vi "Car Data Live.vi"(1 "Input Array":string[](array[string])) -> (0 "CAR DATA":T1)   [LabVIEW 2014]
uses:
  Type Def/CAR Data Cluster.ctl
  Type Def/CAN Message Live.ctl
panel:
  out "Time Size":i32
  out "Time":dbl[](array[numeric]) format="%.2f"
  out "DECAYIGN(+) - DECAYIGN(-)":dbl
  out "DECAYINJ(+) - DECAYINJ(-)":dbl
  out "DTPS-":dbl
  out "DTPS+":dbl
  out "Speed 2":dbl
  out "Speed 1":dbl
  out "Phase High":dbl
  out "Phase Low":dbl
  out "Spark 1":dbl
  out "Inj Low":dbl
  out "K Lambda 2":dbl
  out "K Lambda 1":dbl
  out "Lambda 2 AVG":dbl
  out "Lambda 2 RAW":dbl
  out "Lambda 1 RAW":dbl
  out "Lambda 1 AVG":dbl
  out "BAR0":u32
  out "VBB 3":dbl
  out "VBB 2":dbl
  out "VBB 1":dbl
  out "T Oil":u32
  out "T Air":i32
  out "T H20":i32
  out "map":u32
  out "TPS":dbl
  out "rev/min":u32
  out "revs":u32
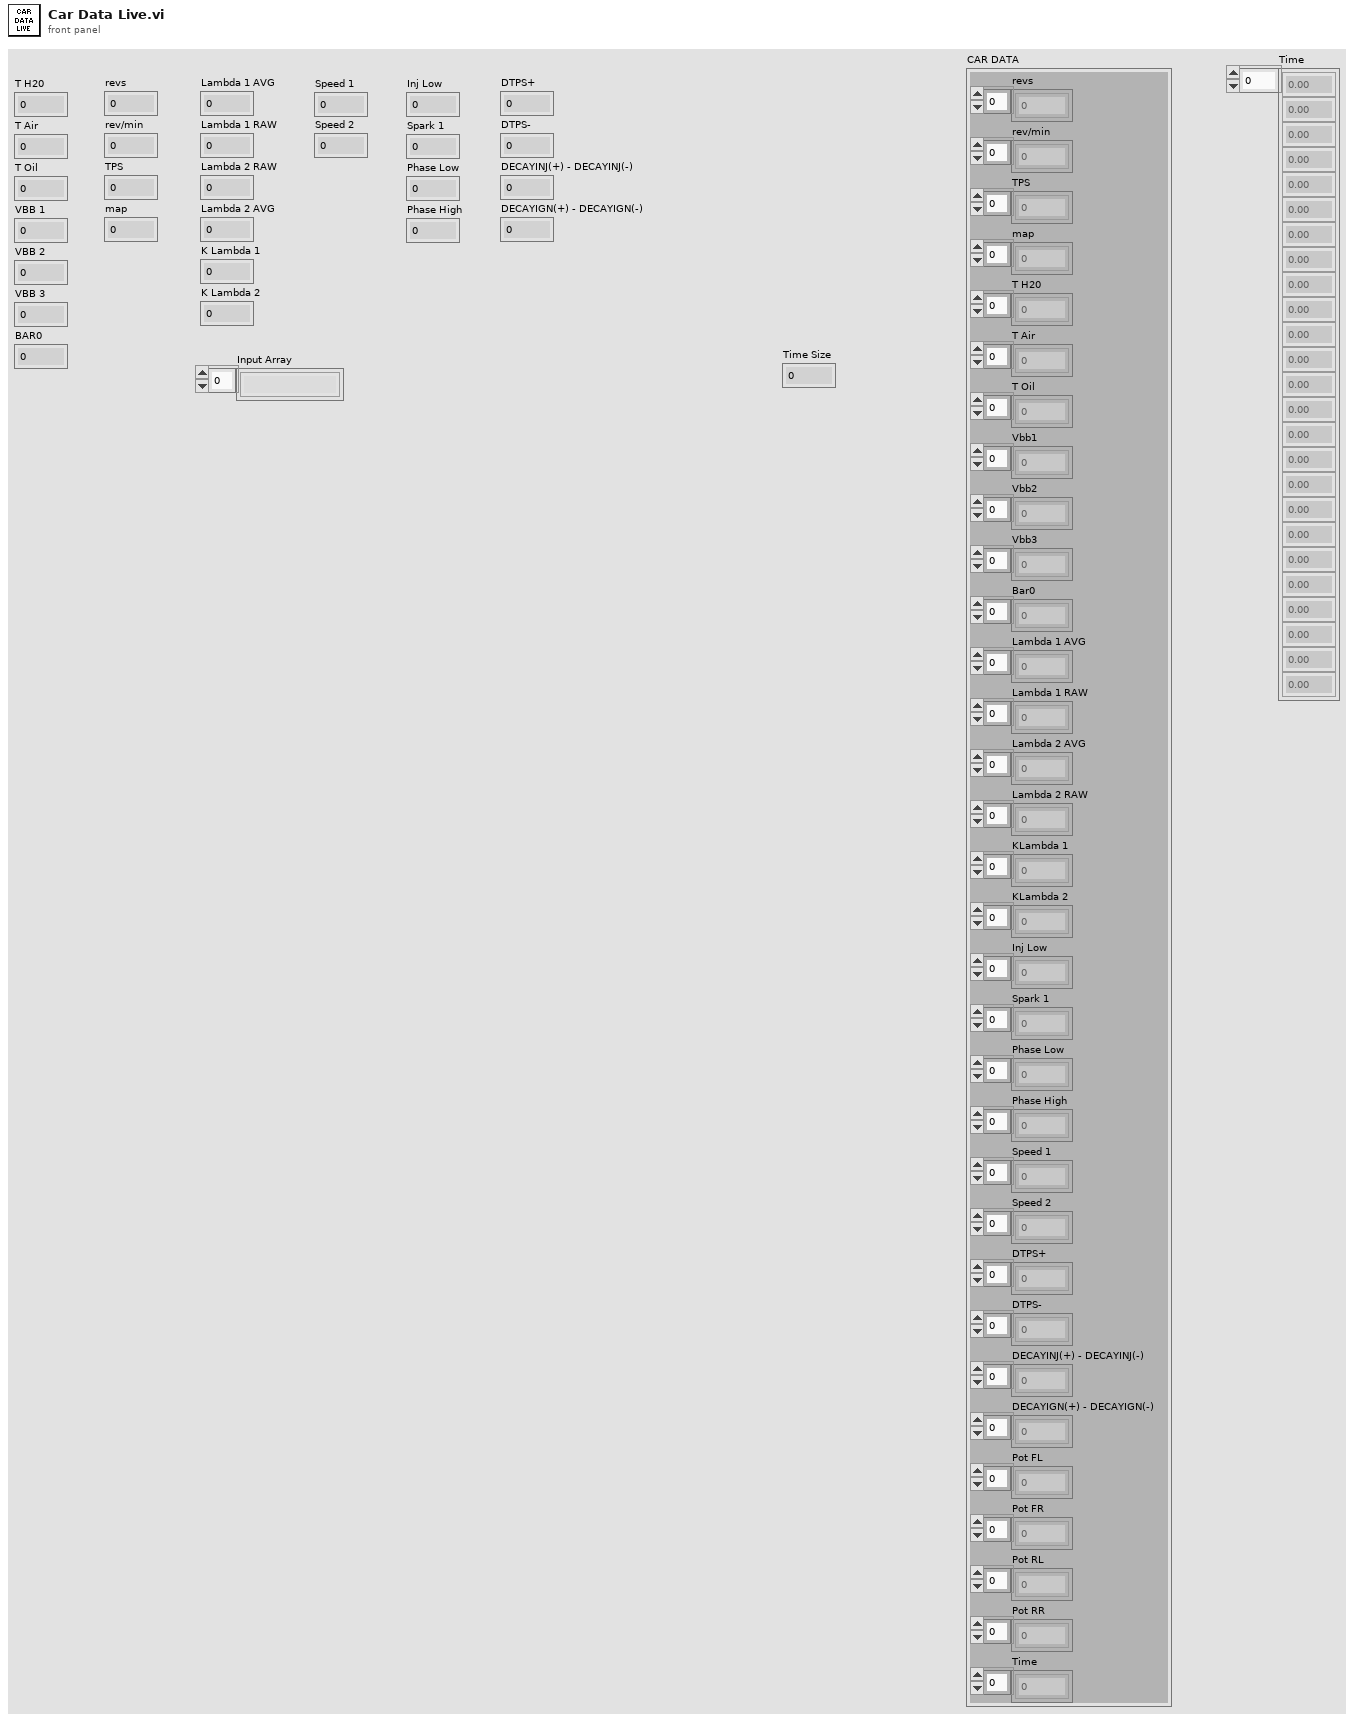
[diagram p1: front panel]
types:
  T1 = typedef "CAR Data Cluster.ctl" = cluster{"revs":dbl[], "rev/min":dbl[], "TPS":dbl[], "map":dbl[], "T H20":dbl[], "T Air":dbl[], "T Oil":dbl[], "Vbb1":dbl[], "Vbb2":dbl[], "Vbb3":dbl[], "Bar0":dbl[], "Lambda 1 AVG":dbl[], "Lambda 1 RAW":dbl[], "Lambda 2 AVG":dbl[], "Lambda 2 RAW":dbl[], "KLambda 1":dbl[], "KLambda 2":dbl[], "Inj Low":dbl[], "Spark 1":dbl[], "Phase Low":dbl[], "Phase High":dbl[], "Speed 1":dbl[], "Speed 2":dbl[], "DTPS+":dbl[], "DTPS-":dbl[], "DECAYINJ(+) - DECAYINJ(-)":dbl[], "DECAYIGN(+) - DECAYIGN(-)":dbl[], "Pot FL":dbl[], "Pot FR":dbl[], "Pot RL":dbl[], "Pot RR":dbl[], "Time":dbl[]}
  T2 = cluster{"revs":dbl[], "rev/min":dbl[], "TPS":dbl[], "map":dbl[], "T H20":dbl[], "T Air":dbl[], "T Oil":dbl[], "Vbb1":dbl[], "Vbb2":dbl[], "Vbb3":dbl[], "Bar0":dbl[], "Lambda 1 AVG":dbl[], "Lambda 1 RAW":dbl[], "Lambda 2 AVG":dbl[], "Lambda 2 RAW":dbl[], "KLambda 1":dbl[], "KLambda 2":dbl[], "Inj Low":dbl[], "Spark 1":dbl[], "Phase Low":dbl[], "Phase High":dbl[], "Speed 1":dbl[], "Speed 2":dbl[], "DTPS+":dbl[], "DTPS-":dbl[], "DECAYINJ(+) - DECAYINJ(-)":dbl[], "DECAYIGN(+) - DECAYIGN(-)":dbl[], "Pot FL":dbl[], "Pot FR":dbl[], "Pot RL":dbl[], "Pot RR":dbl[], "Time":dbl[]}
  T3 = typedef "CAN Message Live.ctl" = cluster{"Time Dif.":i32, "ID":i32, "Message":string}
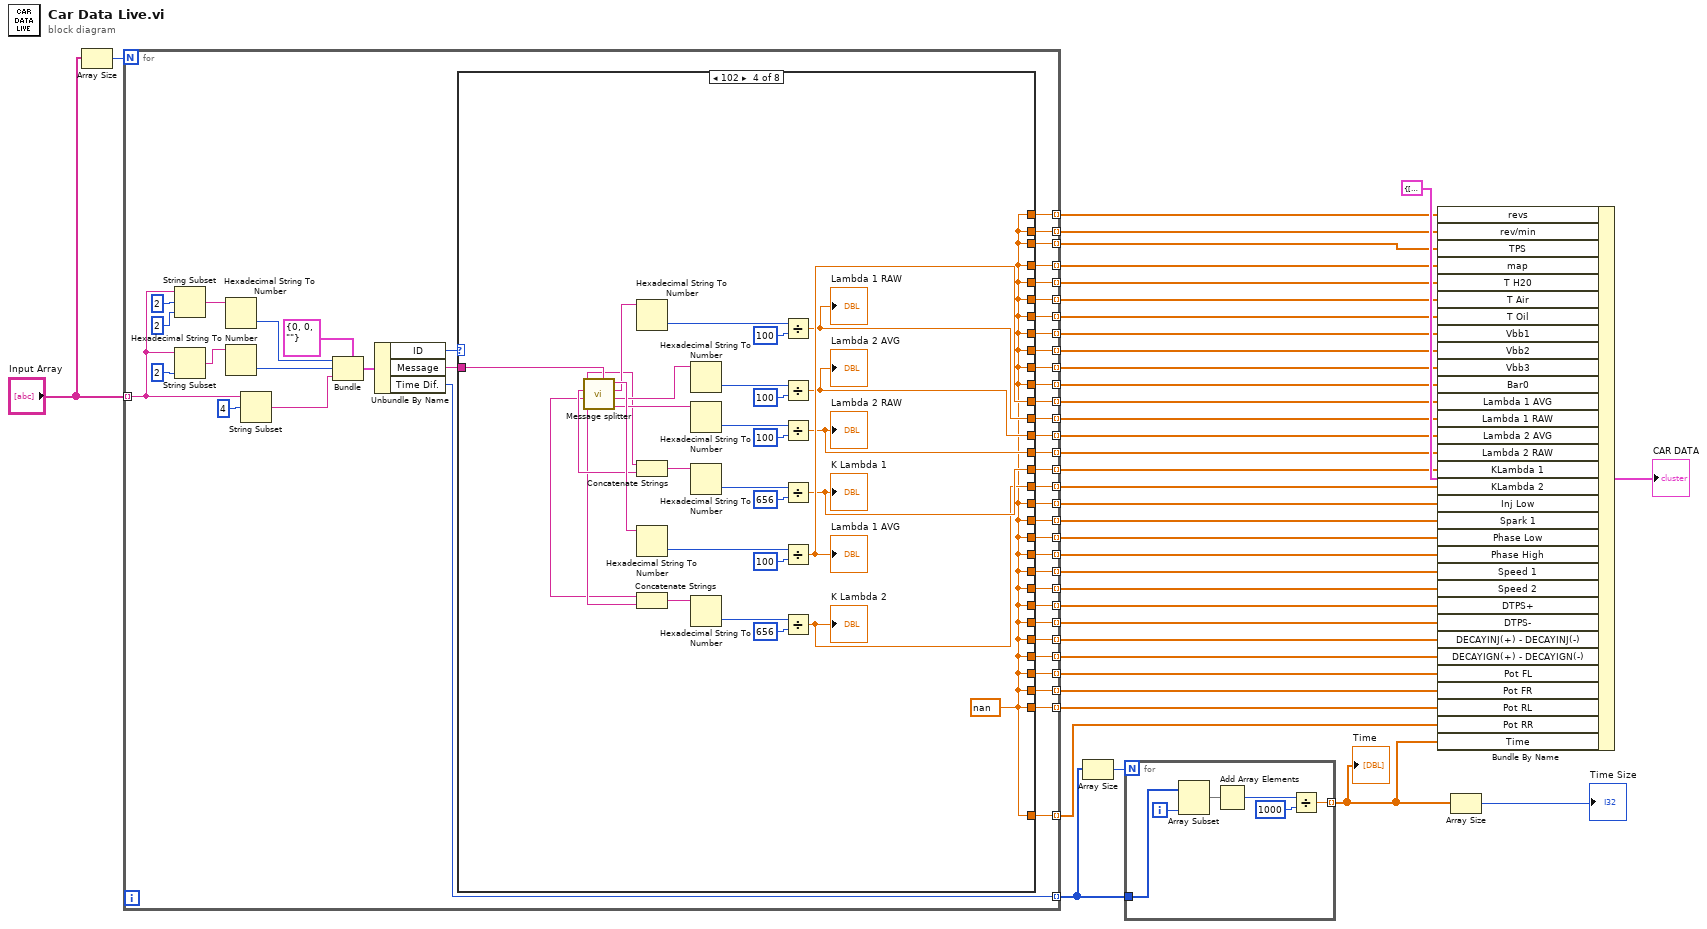
[diagram p0: block diagram]
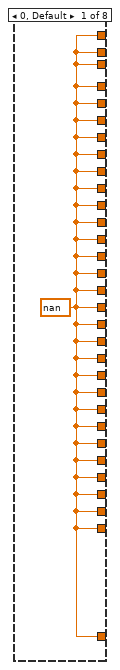
[diagram p2: hidden frame]
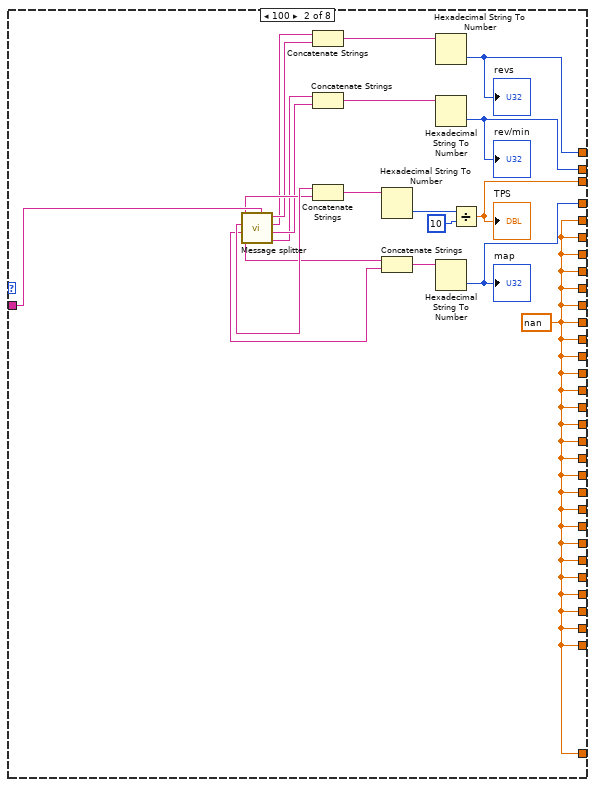
[diagram p3: hidden frame]
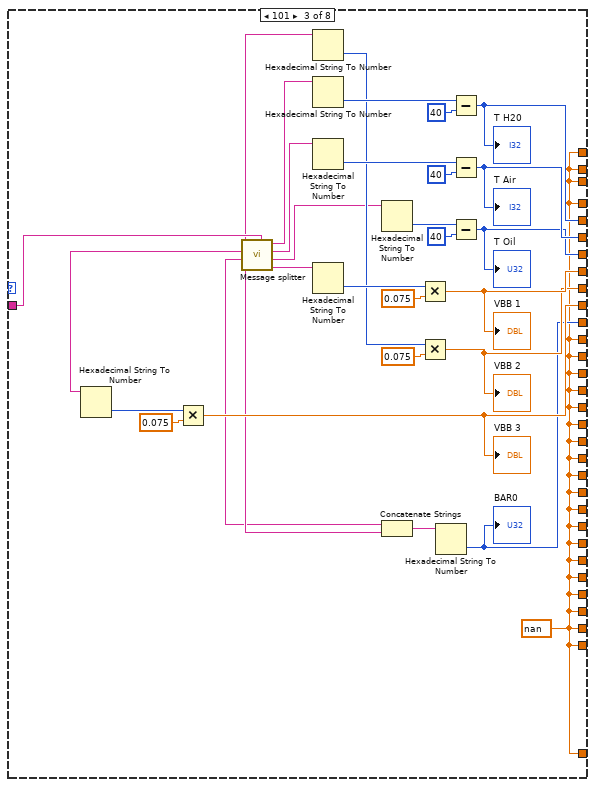
[diagram p4: hidden frame]
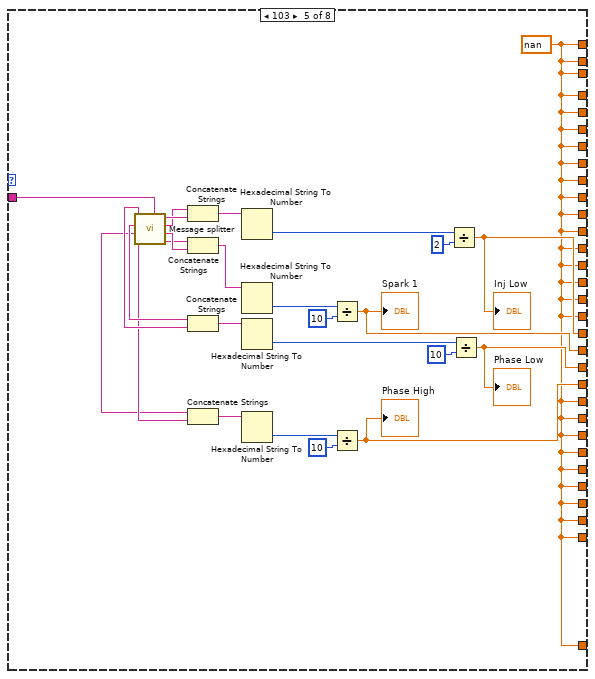
[diagram p5: hidden frame]
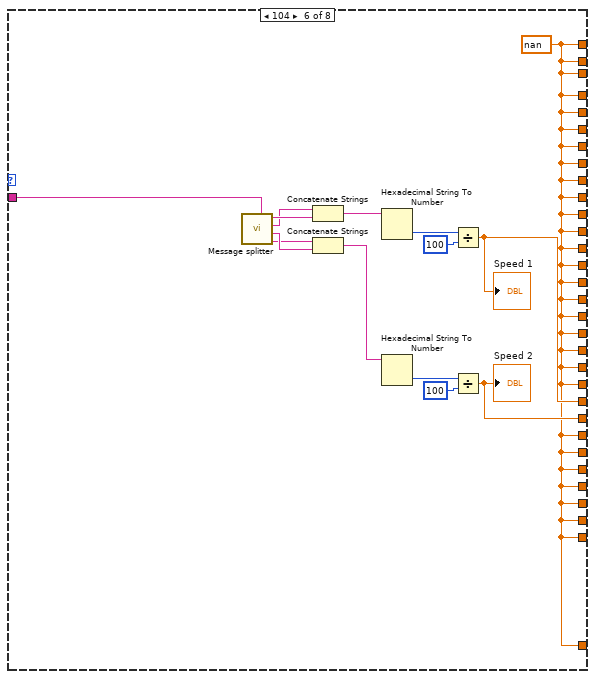
[diagram p6: hidden frame]
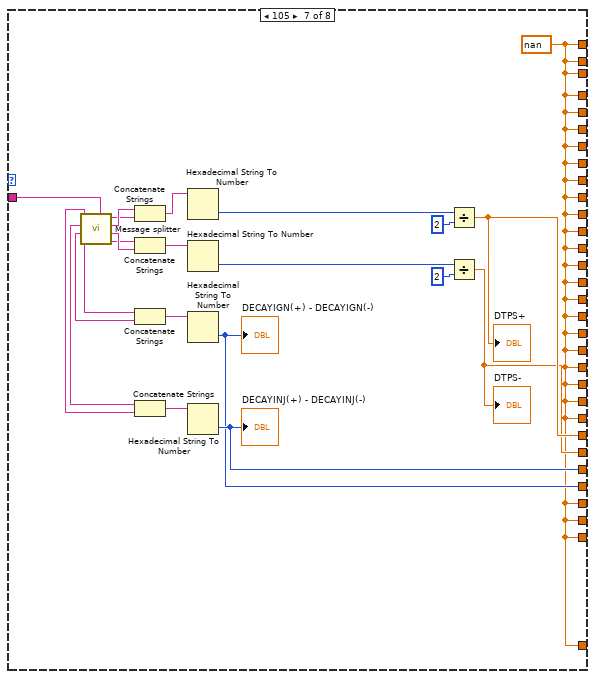
[diagram p7: hidden frame]
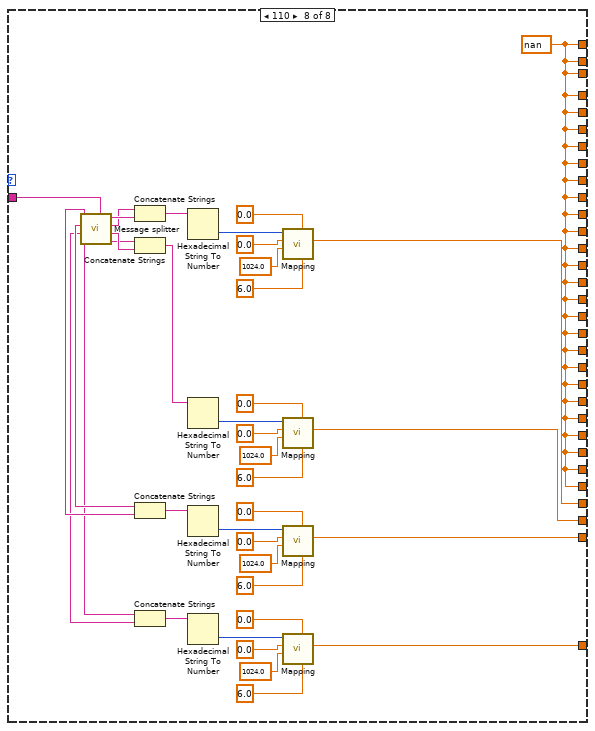
[diagram p8: hidden frame]
diagram:
  n1 = Array Size(array="Input Array") -> (size(s)=w2:i32)
  n2 = for {
    N: w2 -> [_]
    tunnel: [w82] -> w39 mode=indexing
    tunnel: [w81] -> w34 mode=indexing
    tunnel: [w80] -> w36 mode=indexing
    tunnel: [w79] -> w35 mode=indexing
    tunnel: [w78] -> w33 mode=indexing
    tunnel: [w77] -> w32 mode=indexing
    tunnel: [w76] -> w31 mode=indexing
    tunnel: [w75] -> w30 mode=indexing
    tunnel: [w74] -> w29 mode=indexing
    tunnel: [w73] -> w28 mode=indexing
    tunnel: [w72] -> w27 mode=indexing
    tunnel: [w71] -> w26 mode=indexing
    tunnel: [w70] -> w25 mode=indexing
    tunnel: [w69] -> w24 mode=indexing
    tunnel: [w68] -> w23 mode=indexing
    tunnel: [w67] -> w22 mode=indexing
    tunnel: [w66] -> w21 mode=indexing
    tunnel: [w65] -> w20 mode=indexing
    tunnel: [w64] -> w19 mode=indexing
    tunnel: [w63] -> w18 mode=indexing
    tunnel: [w62] -> w17 mode=indexing
    tunnel: [w61] -> w16 mode=indexing
    tunnel: [w60] -> w15 mode=indexing
    tunnel: [w59] -> w14 mode=indexing
    tunnel: [w58] -> w13 mode=indexing
    tunnel: [w57] -> w12 mode=indexing
    tunnel: [w56] -> w11 mode=indexing
    tunnel: [w55] -> w10 mode=indexing
    tunnel: [w54] -> w9 mode=indexing
    tunnel: [w53] -> w8 mode=indexing
    tunnel: [w52] -> w7 mode=indexing
    tunnel: [w51] -> w6 mode=indexing
    tunnel: "Input Array" -> [w44] mode=indexing
    n3 = String Subset(string=w44, offset (0)=2, length (rest)=2 ("length (rest)")) -> (substring=w46:string)
    n4 = String Subset(string=w44, length (rest)=2 ("length (rest)")) -> (substring=w50:string)  [unwired: 1 in]
    n5 = Hexadecimal String To Number(string=w46) -> (number=w42:u32)  [unwired: 2 in, 1 out]
    n6 = Hexadecimal String To Number(string=w50) -> (number=w43:u32)  [unwired: 2 in, 1 out]
    n7 = String Subset(string=w44, offset (0)=4) -> (substring=w41:string)  [unwired: 1 in]
    n8 = Bundle(cluster=T3 {"Time Dif."=0, "ID"=0, "Message"=""} ("Cluster"), "Time Dif."=w42, "ID"=w43, "Message"=w41) -> (w85:T3)
    n9 = Unbundle By Name(w85) -> ("ID"=w84:i32, "Message"=w83:string, "Time Dif."=w82:i32)
    n10 = case shown="102" w84 {
      tunnel: w83 -> [_ w100 w123 w166 w192 w206 w228 w266]
      tunnel: [w86 w99 w107 w137 w167 w193 w207 w265] -> w81
      tunnel: [w86 w98 w107 w137 w167 w193 w207 w265] -> w80
      tunnel: [w86 w97 w107 w137 w167 w193 w207 w265] -> w79
      tunnel: [w86 w96 w107 w137 w167 w193 w207 w265] -> w78
      tunnel: [w86 w87 w116 w137 w167 w193 w207 w265] -> w77
      tunnel: [w86 w87 w115 w137 w167 w193 w207 w265] -> w76
      tunnel: [w86 w87 w114 w137 w167 w193 w207 w265] -> w75
      tunnel: [w86 w87 w113 w137 w167 w193 w207 w265] -> w74
      tunnel: [w86 w87 w112 w137 w167 w193 w207 w265] -> w73
      tunnel: [w86 w87 w111 w137 w167 w193 w207 w265] -> w72
      tunnel: [w86 w87 w110 w137 w167 w193 w207 w265] -> w71
      tunnel: [w86 w87 w107 w145 w167 w193 w207 w265] -> w70
      tunnel: [w86 w87 w107 w144 w167 w193 w207 w265] -> w69
      tunnel: [w86 w87 w107 w143 w167 w193 w207 w265] -> w68
      tunnel: [w86 w87 w107 w142 w167 w193 w207 w265] -> w67
      tunnel: [w86 w87 w107 w141 w167 w193 w207 w265] -> w66
      tunnel: [w86 w87 w107 w140 w167 w193 w207 w265] -> w65
      tunnel: [w86 w87 w107 w137 w179 w193 w207 w265] -> w64
      tunnel: [w86 w87 w107 w137 w178 w193 w207 w265] -> w63
      tunnel: [w86 w87 w107 w137 w177 w193 w207 w265] -> w62
      tunnel: [w86 w87 w107 w137 w176 w193 w207 w265] -> w61
      tunnel: [w86 w87 w107 w137 w167 w199 w207 w265] -> w60
      tunnel: [w86 w87 w107 w137 w167 w198 w207 w265] -> w59
      tunnel: [w86 w87 w107 w137 w167 w193 w219 w265] -> w58
      tunnel: [w86 w87 w107 w137 w167 w193 w218 w265] -> w57
      tunnel: [w86 w87 w107 w137 w167 w193 w217 w265] -> w56
      tunnel: [w86 w87 w107 w137 w167 w193 w216 w265] -> w55
      tunnel: [w86 w87 w107 w137 w167 w193 w207 w256] -> w54
      tunnel: [w86 w87 w107 w137 w167 w193 w207 w247] -> w53
      tunnel: [w86 w87 w107 w137 w167 w193 w207 w230] -> w52
      tunnel: [w86 w87 w107 w137 w167 w193 w207 w229] -> w51
      frame 0, Default {
        w86 = nan
      }
      frame 100 {
        w87 = nan
        n11 = call "Message splitter.vi"("Message in"=w100) -> ("Byte 4"=w90:string, "Byte 3"=w91:string, "Byte 2"=w92:string, "Byte 1"=w93:string, "Byte 8"=w88:string, "Byte 7"=w89:string, "Byte 6"=w95:string, "Byte 5"=w94:string)  [unwired: 3 in]
        n12 = Concatenate Strings(w92, w93) -> (w106:string)
        n13 = Concatenate Strings(w90, w91) -> (w105:string)
        n14 = Concatenate Strings(w95, w94) -> (w104:string)
        n15 = Hexadecimal String To Number(string=w104) -> (number=w103:u32)  [unwired: 2 in, 1 out]
        n16 = Concatenate Strings(w88, w89) -> (w101:string)
        n17 = Hexadecimal String To Number(string=w106) -> (number=w98:u32)  [unwired: 2 in, 1 out]
        "revs" <- w98
        n18 = Hexadecimal String To Number(string=w105) -> (number=w97:u32)  [unwired: 2 in, 1 out]
        "rev/min" <- w97
        n19 = Hexadecimal String To Number(string=w101) -> (number=w96:u32)  [unwired: 2 in, 1 out]
        "map" <- w96
        n20 = Divide(x=w103, y=u32 10) -> (x/y=w99:dbl)
        "TPS" <- w99
      }
      frame 101 {
        w107 = nan
        n21 = call "Message splitter.vi"("Message in"=w123) -> ("Byte 4"=w119:string, "Byte 3"=w120:string, "Byte 2"=w121:string, "Byte 1"=w122:string, "Byte 8"=w109:string, "Byte 7"=w108:string, "Byte 6"=w117:string, "Byte 5"=w118:string)  [unwired: 3 in]
        n22 = Hexadecimal String To Number(string=w117) -> (number=w126:u32)  [unwired: 2 in, 1 out]
        n23 = Multiply(x=w126, y=0.075) -> (x*y=w111:dbl)
        "VBB 3" <- w111
        n24 = Hexadecimal String To Number(string=w118) -> (number=w128:u32)  [unwired: 2 in, 1 out]
        n25 = Hexadecimal String To Number(string=w122) -> (number=w136:u32)  [unwired: 2 in, 1 out]
        n26 = Hexadecimal String To Number(string=w121) -> (number=w133:u32)  [unwired: 2 in, 1 out]
        n27 = Hexadecimal String To Number(string=w119) -> (number=w130:u32)  [unwired: 2 in, 1 out]
        n28 = Hexadecimal String To Number(string=w120) -> (number=w131:u32)  [unwired: 2 in, 1 out]
        n29 = Concatenate Strings(w108, w109) -> (w124:string)
        n30 = Multiply(x=w130, y=0.075) -> (x*y=w113:dbl)
        "VBB 1" <- w113
        n31 = Multiply(x=w128, y=0.075) -> (x*y=w112:dbl)
        "VBB 2" <- w112
        n32 = Hexadecimal String To Number(string=w124) -> (number=w110:u32)  [unwired: 2 in, 1 out]
        "BAR0" <- w110
        n33 = Subtract(x=w136, y=u32 40) -> (x-y=w116:u32)
        "T H20" <- w116
        n34 = Subtract(x=w133, y=u32 40) -> (x-y=w115:u32)
        "T Air" <- w115
        n35 = Subtract(x=w131, y=u32 40) -> (x-y=w114:u32)
        "T Oil" <- w114
      }
      frame 102 {
        w137 = nan
        n36 = call "Message splitter.vi"("Message in"=w166) -> ("Byte 4"=w154:string, "Byte 3"=w155:string, "Byte 2"=w156:string, "Byte 1"=w165:string, "Byte 8"=w139:string, "Byte 7"=w138:string, "Byte 6"=w152:string, "Byte 5"=w153:string)  [unwired: 3 in]
        n37 = Hexadecimal String To Number(string=w156) -> (number=w162:u32)  [unwired: 2 in, 1 out]
        n38 = Concatenate Strings(w153, w152) -> (w149:string)
        n39 = Hexadecimal String To Number(string=w165) -> (number=w164:u32)  [unwired: 2 in, 1 out]
        n40 = Concatenate Strings(w138, w139) -> (w146:string)
        n41 = Hexadecimal String To Number(string=w155) -> (number=w158:u32)  [unwired: 2 in, 1 out]
        n42 = Hexadecimal String To Number(string=w154) -> (number=w160:u32)  [unwired: 2 in, 1 out]
        n43 = Hexadecimal String To Number(string=w149) -> (number=w151:u32)  [unwired: 2 in, 1 out]
        n44 = Hexadecimal String To Number(string=w146) -> (number=w148:u32)  [unwired: 2 in, 1 out]
        n45 = Divide(x=w162, y=u32 100) -> (x/y=w144:dbl)
        "Lambda 1 RAW" <- w144
        n46 = Divide(x=w158, y=u32 100) -> (x/y=w143:dbl)
        "Lambda 2 AVG" <- w143
        n47 = Divide(x=w160, y=u32 100) -> (x/y=w142:dbl)
        "Lambda 2 RAW" <- w142
        n48 = Divide(x=w151, y=u32 656) -> (x/y=w141:dbl)
        "K Lambda 1" <- w141
        n49 = Divide(x=w164, y=u32 100) -> (x/y=w145:dbl)
        "Lambda 1 AVG" <- w145
        n50 = Divide(x=w148, y=u32 656) -> (x/y=w140:dbl)
        "K Lambda 2" <- w140
      }
      frame 103 {
        w167 = nan
        n51 = call "Message splitter.vi"("Message in"=w192) -> ("Byte 4"=w172:string, "Byte 3"=w173:string, "Byte 2"=w174:string, "Byte 1"=w175:string, "Byte 8"=w169:string, "Byte 7"=w168:string, "Byte 6"=w171:string, "Byte 5"=w170:string)  [unwired: 3 in]
        n52 = Concatenate Strings(w174, w175) -> (w191:string)
        n53 = Concatenate Strings(w172, w173) -> (w188:string)
        n54 = Concatenate Strings(w171, w170) -> (w185:string)
        n55 = Concatenate Strings(w168, w169) -> (w182:string)
        n56 = Hexadecimal String To Number(string=w191) -> (number=w190:u32)  [unwired: 2 in, 1 out]
        n57 = Hexadecimal String To Number(string=w188) -> (number=w187:u32)  [unwired: 2 in, 1 out]
        n58 = Hexadecimal String To Number(string=w185) -> (number=w184:u32)  [unwired: 2 in, 1 out]
        n59 = Hexadecimal String To Number(string=w182) -> (number=w181:u32)  [unwired: 2 in, 1 out]
        n60 = Divide(x=w187, y=u32 10) -> (x/y=w178:dbl)
        "Spark 1" <- w178
        n61 = Divide(x=w181, y=u32 10) -> (x/y=w176:dbl)
        "Phase High" <- w176
        n62 = Divide(x=w190, y=u32 2) -> (x/y=w179:dbl)
        "Inj Low" <- w179
        n63 = Divide(x=w184, y=u32 10) -> (x/y=w177:dbl)
        "Phase Low" <- w177
      }
      frame 104 {
        w193 = nan
        n64 = call "Message splitter.vi"("Message in"=w206) -> ("Byte 4"=w194:string, "Byte 3"=w195:string, "Byte 2"=w196:string, "Byte 1"=w197:string)  [unwired: 3 in, 4 out]
        n65 = Concatenate Strings(w196, w197) -> (w205:string)
        n66 = Concatenate Strings(w194, w195) -> (w200:string)
        n67 = Hexadecimal String To Number(string=w205) -> (number=w204:u32)  [unwired: 2 in, 1 out]
        n68 = Hexadecimal String To Number(string=w200) -> (number=w202:u32)  [unwired: 2 in, 1 out]
        n69 = Divide(x=w204, y=u32 100) -> (x/y=w199:dbl)
        "Speed 1" <- w199
        n70 = Divide(x=w202, y=u32 100) -> (x/y=w198:dbl)
        "Speed 2" <- w198
      }
      frame 105 {
        w207 = nan
        n71 = call "Message splitter.vi"("Message in"=w228) -> ("Byte 4"=w212:string, "Byte 3"=w213:string, "Byte 2"=w215:string, "Byte 1"=w214:string, "Byte 8"=w209:string, "Byte 7"=w208:string, "Byte 6"=w210:string, "Byte 5"=w211:string)  [unwired: 3 in]
        n72 = Concatenate Strings(w215, w214) -> (w227:string)
        n73 = Concatenate Strings(w212, w213) -> (w224:string)
        n74 = Concatenate Strings(w209, w208) -> (w220:string)
        n75 = Concatenate Strings(w210, w211) -> (w221:string)
        n76 = Hexadecimal String To Number(string=w227) -> (number=w226:u32)  [unwired: 2 in, 1 out]
        n77 = Hexadecimal String To Number(string=w224) -> (number=w223:u32)  [unwired: 2 in, 1 out]
        n78 = Hexadecimal String To Number(string=w220) -> (number=w216:u32)  [unwired: 2 in, 1 out]
        "DECAYIGN(+) - DECAYIGN(-)" <- w216
        n79 = Hexadecimal String To Number(string=w221) -> (number=w217:u32)  [unwired: 2 in, 1 out]
        "DECAYINJ(+) - DECAYINJ(-)" <- w217
        n80 = Divide(x=w226, y=u32 2) -> (x/y=w219:dbl)
        "DTPS+" <- w219
        n81 = Divide(x=w223, y=u32 2) -> (x/y=w218:dbl)
        "DTPS-" <- w218
      }
      frame 110 {
        w265 = nan
        n82 = call "Message splitter.vi"("Message in"=w266) -> ("Byte 4"=w248:string, "Byte 3"=w249:string, "Byte 2"=w263:string, "Byte 1"=w264:string, "Byte 8"=w232:string, "Byte 7"=w231:string, "Byte 6"=w233:string, "Byte 5"=w234:string)  [unwired: 3 in]
        n83 = Concatenate Strings(w263, w264) -> (w262:string)
        n84 = Concatenate Strings(w248, w249) -> (w255:string)
        n85 = Concatenate Strings(w233, w234) -> (w246:string)
        n86 = Concatenate Strings(w232, w231) -> (w240:string)
        n87 = Hexadecimal String To Number(string=w262) -> (number=w261:u32)  [unwired: 2 in, 1 out]
        n88 = Hexadecimal String To Number(string=w255) -> (number=w254:u32)  [unwired: 2 in, 1 out]
        n89 = Hexadecimal String To Number(string=w246) -> (number=w245:u32)  [unwired: 2 in, 1 out]
        n90 = Hexadecimal String To Number(string=w240) -> (number=w239:u32)  [unwired: 2 in, 1 out]
        n91 = call "Mapping.vi"("out_max"=6.0, "out_min"=0.0, "in_max"=1024.0, "in_min"=0.0, "x"=w261) -> ("y"=w256:dbl)  [unwired: 6 in]
        n92 = call "Mapping.vi"("out_max"=6.0, "out_min"=0.0, "in_max"=1024.0, "in_min"=0.0, "x"=w254) -> ("y"=w247:dbl)  [unwired: 6 in]
        n93 = call "Mapping.vi"("out_max"=6.0, "out_min"=0.0, "in_max"=1024.0, "in_min"=0.0, "x"=w245) -> ("y"=w230:dbl)  [unwired: 6 in]
        n94 = call "Mapping.vi"("out_max"=6.0, "out_min"=0.0, "in_max"=1024.0, "in_min"=0.0, "x"=w239) -> ("y"=w229:dbl)  [unwired: 6 in]
      }
    }
  }
  n95 = Array Size(array=w39) -> (size(s)=w38:i32)
  n96 = for {
    N: w38 -> [_]
    tunnel: w39 -> [w272]
    tunnel: [w267] -> w4 mode=indexing
    i -> [w271]
    n97 = Array Subset(array=w272, length=w271) -> (w270:i32[])  [unwired: 1 in]
    n98 = Add Array Elements(numeric array=w270) -> (sum=w269:i32)
    n99 = Divide(x=w269, y=1000) -> (x/y=w267:dbl)
  }
  "Time" <- w4
  n100 = Bundle By Name(cluster=T2 {"revs"=[], "rev/min"=[], "TPS"=[], "map"=[], "T H20"=[], "T Air"=[], "T Oil"=[], "Vbb1"=[], "Vbb2"=[], "Vbb3"=[], "Bar0"=[], "Lambda 1 AVG"=[], "Lambda 1 RAW"=[], "Lambda 2 AVG"=[], "Lambda 2 RAW"=[], "KLambda 1"=[], "KLambda 2"=[], "Inj Low"=[], "Spark 1"=[], "Phase Low"=[], "Phase High"=[], "Speed 1"=[], "Speed 2"=[], "DTPS+"=[], "DTPS-"=[], "DECAYINJ(+) - DECAYINJ(-)"=[], "DECAYIGN(+) - DECAYIGN(-)"=[], "Pot FL"=[], "Pot FR"=[], "Pot RL"=[], "Pot RR"=[], "Time"=[]}, "revs"=w36, "rev/min"=w35, "TPS"=w34, "map"=w33, "T H20"=w32, "T Air"=w31, "T Oil"=w30, "Vbb1"=w29, "Vbb2"=w28, "Vbb3"=w27, "Bar0"=w26, "Lambda 1 AVG"=w25, "Lambda 1 RAW"=w24, "Lambda 2 AVG"=w23, "Lambda 2 RAW"=w22, "KLambda 1"=w21, "KLambda 2"=w20, "Inj Low"=w19, "Spark 1"=w18, "Phase Low"=w17, "Phase High"=w16, "Speed 1"=w15, "Speed 2"=w14, "DTPS+"=w13, "DTPS-"=w12, "DECAYINJ(+) - DECAYINJ(-)"=w11, "DECAYIGN(+) - DECAYIGN(-)"=w10, "Pot FL"=w9, "Pot FR"=w8, "Pot RL"=w7, "Pot RR"=w6, "Time"=w4) -> (→"CAR DATA":T2)
  n101 = Array Size(array=w4) -> (size(s)=→"Time Size":i32)
